vi "LoopStatus.vi"(7 "Numeric":i32, 8 "error in (no error)":errorcluster, 9 "Status":bool, 10 "Loop in":T1, 11 "Finished Late? [i-1]":bool) -> (1 "error out":errorcluster, 2 "status":bool, 3 "Loop out":T1)   [LabVIEW 2018, in "SubVi.lvlib"]
uses:
  SubVi.lvlib
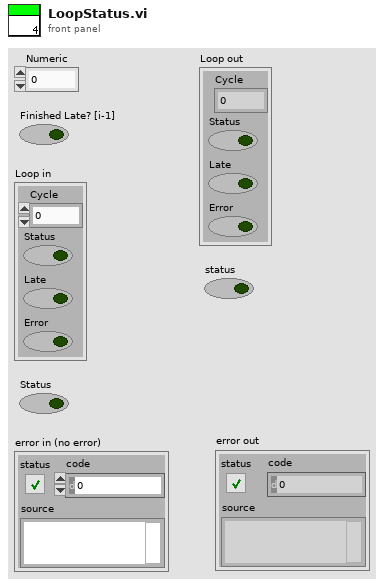
[diagram p1: front panel]
types:
  T1 = cluster{"Cycle":i32, "Status":bool, "Late":bool, "Error":bool}
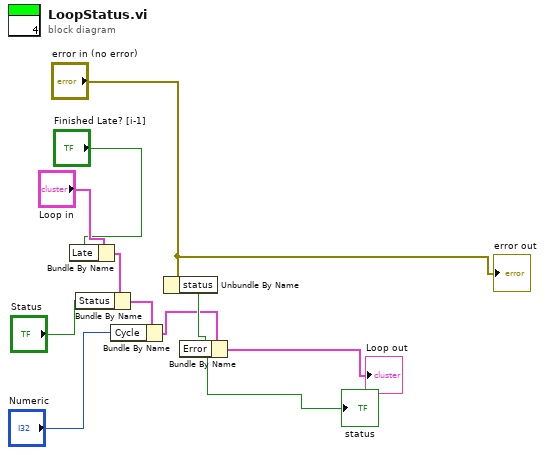
[diagram p0: block diagram]
diagram:
  n1 = Bundle By Name(cluster="Loop in", "Late"="Finished Late? [i-1]") -> (w5:T1)
  n2 = Bundle By Name(cluster=w5, "Status"="Status") -> (w6:T1)
  n3 = Bundle By Name(cluster=w6, "Cycle"="Numeric") -> (w7:T1)
  n4 = Unbundle By Name("error in (no error)") -> ("status"=w10:bool)
  "status" <- w10
  n5 = Bundle By Name(cluster=w7, "Error"=w10) -> (→"Loop out":T1)
  "error out" <- "error in (no error)"
